vi "Type Paths.vi"(8 "error in (no error)":errorcluster, 11 "Editor in":refnum<class "Entity Editor.lvclass">) -> (0 "error out":errorcluster, 3 "Editor out":refnum<class "Entity Editor.lvclass">)   [LabVIEW 2020, in "Conditum-Tools.lvlib" / "Entity Editor.lvclass"]
uses:
  Entity Editor.lvclass
  Entity Editor.lvclass/Entity Editor.ctl
  25459f78-de0e-4e63-8b90-971e39c3733c.vi
  d3a34e09-33f2-4a0f-81e0-cc7ce0d6e4e0.vi
  Type Paths OoC.vi
  Editor Context.vi
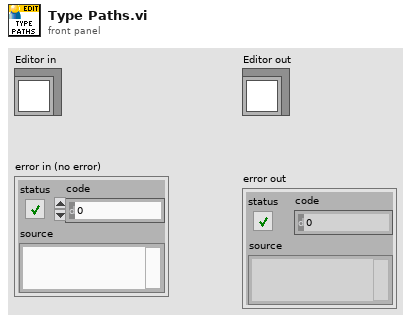
[diagram p1: front panel]
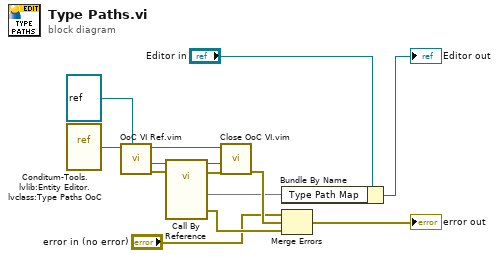
[diagram p0: block diagram]
diagram:
  n1 = vi-ref "Conditum-Tools.lvlib:Entity Editor.lvclass:Type Paths OoC.vi"() -> (w2:refnum<vi>)
  n2 = call "OoC VI Ref.vim"("VI Type"=refnum<vi> refnum, "OoC SVR"=w2) -> ("error out"=w7:errorcluster, "vi reference"=w8:refnum<vi>, "context"=w4:refnum<vi>)  [unwired: 7 in]
  n3 = call-by-ref "?"(reference=w8, error in=w7) -> (reference out=w5:refnum<vi>, error out=w6:errorcluster, 0:"error out"=w13:errorcluster, "Type Path Map"=w10:map{path, path})  [unwired: 10 in]
  n4 = call "Close OoC VI.vim"("error in (no error)"=w6, "vi reference"=w5, "context"=w4) -> ("error out"=w14:errorcluster)  [unwired: 8 in]
  n5 = Bundle By Name(cluster="Editor in", "Type Path Map"=w10) -> (→"Editor out":refnum<class "Entity Editor.lvclass">)
  n6 = Merge Errors("error in (no error)", w14, w13) -> (→"error out":errorcluster)
